vi "Option Parser.vi"(0 "Yokogawa WT500 in":refnum<class "Yokogawa WT500.lvclass">, 1 "ID":string, 2 "THD?":bool, 3 "Number of Cards":dbl, 4 "ID cluster.Model":string, 5 "error in (no error)":errorcluster, 7 "Option":string) -> (14 "Yokogawa WT500 out":refnum<class "Yokogawa WT500.lvclass">, 19 "error out":errorcluster)   [LabVIEW 2013, in "Universal Power Meter.lvlib" / "Yokogawa WT500.lvlib" / "Yokogawa WT500.lvclass"]
uses:
  Yokogawa WT500.lvclass
  Universal Power Meter class/Universal Power Meter.lvclass
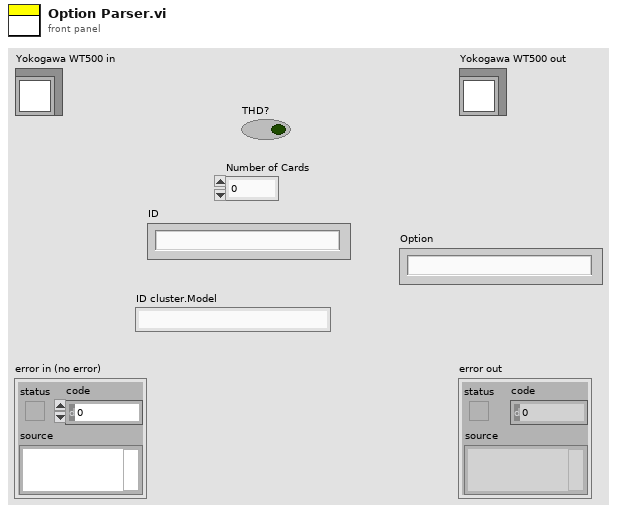
[diagram p1: front panel]
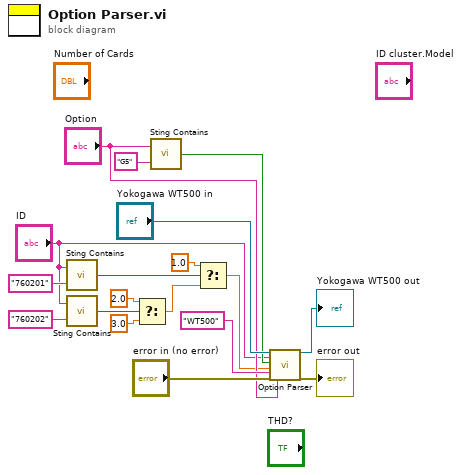
[diagram p0: block diagram]
diagram:
  n1 = call "Sting Contains.vi"("Expression to evaluate"="760201", "Input String"="ID") -> ("Boolean"=w9:bool)
  n2 = call "Sting Contains.vi"("Expression to evaluate"="760202", "Input String"="ID") -> ("Boolean"=w5:bool)
  n3 = Select(t=2.0, s=w5, f=3.0) -> (s? t:f=w4:dbl)
  n4 = call "Sting Contains.vi"("Expression to evaluate"="G5", "Input String"="Option") -> ("Boolean"=w11:bool)
  n5 = Select(t=1.0, s=w9, f=w4) -> (s? t:f=w3:dbl)
  n6 = call-parent "Option Parser.vi"("Universal Power Meter in"="Yokogawa WT500 in", "ID"="ID", "THD?"=w11, "Number of Cards"=w3, "ID cluster.Model"="WT500", "error in (no error)"="error in (no error)", "Option"="Option") -> ("Universal Power Meter out"=→"Yokogawa WT500 out":refnum<class "Yokogawa WT500.lvclass">, "error out"=→"error out":errorcluster)  [unwired: 11 in]
